vi "UTM To Image.vi"(0 "UTM Location":T1, 1 "Image Descriptor":T2={"Upper-Left Corner Coordinates"={"UTM Zone"=0.0, "Hemisphere"=enum."North", "East"=0.0, "North"=0.0}, "Meters/Pixel"=42.294203}, 2 "error in":errorcluster) -> (3 "X":i32, 4 "Y":i32, 5 "Coordinate Outside Image":bool, 6 "error out":errorcluster)   [LabVIEW 2011]
uses:
  0-Image Descriptor.ctl
  2-Think/2 Typedefs/UTM Location.ctl
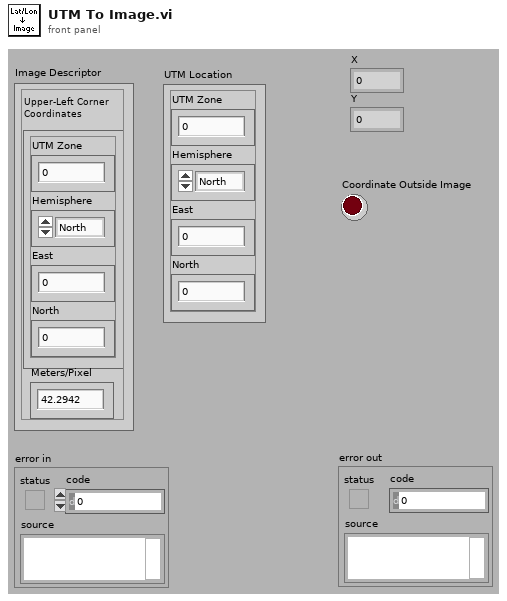
[diagram p1: front panel]
types:
  T1 = typedef "UTM Location.ctl" = cluster{"UTM Zone":dbl, "Hemisphere":enum16{"North", "South"}, "East":dbl, "North":dbl}
  T2 = typedef "0-Image Descriptor.ctl" = cluster{"Upper-Left Corner Coordinates":T1, "Meters/Pixel":dbl}
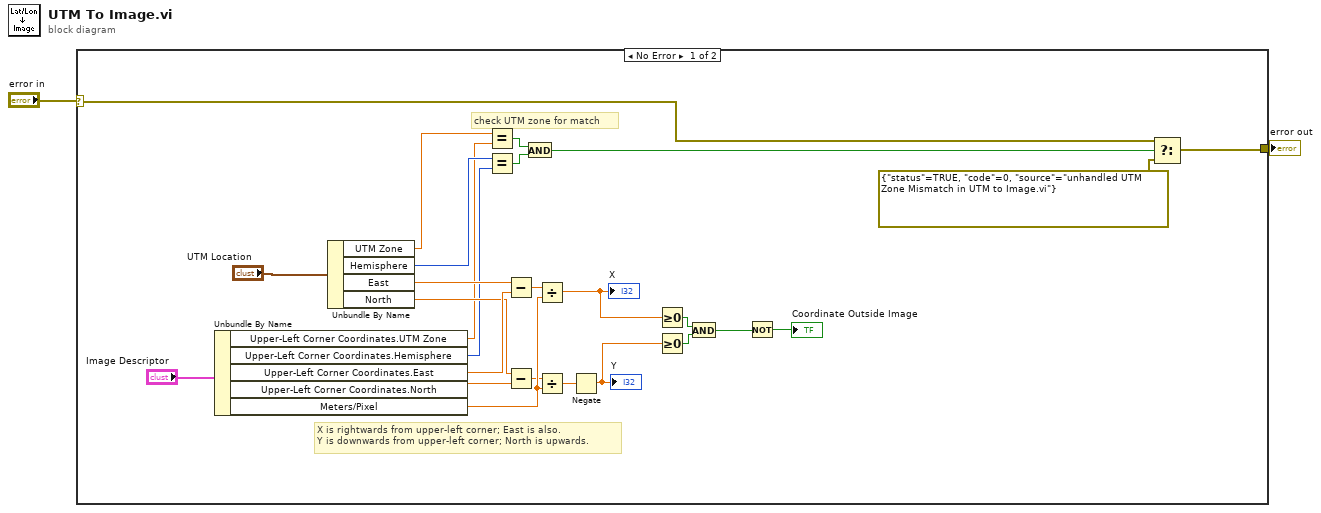
[diagram p0: block diagram]
diagram:
  n1 = case shown="No Error" "error in" {
    selector: "error in" -> [w4 w29]
    tunnel: [w10 w29] -> w1
    frame No Error {
      # "check UTM zone for match"
      # "X is rightwards from upper-left corner; East is also.\nY is downwards from upper-left corner; North is upwards."
      n2 = Unbundle By Name("Image Descriptor") -> ("Upper-Left Corner Coordinates.UTM Zone"=w16:dbl, "Upper-Left Corner Coordinates.Hemisphere"=w17:enum16{"North", "South"}, "Upper-Left Corner Coordinates.East"=w26:dbl, "Upper-Left Corner Coordinates.North"=w25:dbl, "Meters/Pixel"=w24:dbl)
      n3 = Unbundle By Name("UTM Location") -> ("UTM Zone"=w15:dbl, "Hemisphere"=w18:enum16{"North", "South"}, "East"=w21:dbl, "North"=w20:dbl)
      n4 = Equal?(x=w15, y=w16) -> (x = y?=w14:bool)
      n5 = Equal?(x=w18, y=w17) -> (x = y?=w13:bool)
      n6 = Subtract(x=w21, y=w26) -> (x-y=w19:dbl)
      n7 = Subtract(x=w20, y=w25) -> (x-y=w23:dbl)
      n8 = And(x=w14, y=w13) -> (x .and. y?=w12:bool)
      n9 = Divide(x=w19, y=w24) -> (x/y=w9:dbl)
      "X" <- w9
      n10 = Divide(x=w23, y=w24) -> (x/y=w28:dbl)
      n11 = Negate(x=w28) -> (-x=w8:dbl)
      "Y" <- w8
      n12 = Greater Or Equal To 0?(x=w9) -> (x >= 0?=w6:bool)
      n13 = Greater Or Equal To 0?(x=w8) -> (x >= 0?=w7:bool)
      n14 = And(x=w6, y=w7) -> (x .and. y?=w5:bool)
      n15 = Not(x=w5) -> (.not. x?=→"Coordinate Outside Image":bool)
      n16 = Select(t=w4, s=w12, f=errorcluster {"status"=TRUE, "code"=0, "source"="unhandled UTM Zone Mismatch in UTM to Image.vi"} ("error IO")) -> (s? t:f=w10:errorcluster)
    }
    frame Error {
    }
  }
  "error out" <- w1
